vi "Scope_V3.vi"(9 "ObjectChoice":i32[](listbox), 11 "btnSelectObject":bool) -> (0 "strObjectDispArray":string[](array[string]), 1 "mu08ArrayIndexFinalOut":u8[](array[numeric]), 2 "NamePic":picture, 3 "mbfObjectChoiceArray":bool[](array[boolean]))   [LabVIEW 2011]
uses:
  <vilib>/Utility/miscctls.llb/LVPoint32TypeDef.ctl
  GlobalVariable/strGlobalVariable.vi
panel:
  out "mbfStartDraw":bool
  out "btnSelectObject.Txt":string
  out "坐标":T1
  out "mu08ObjectArraySize":u8
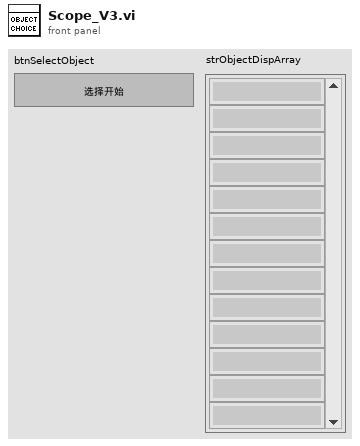
[diagram p1: front panel]
types:
  T1 = typedef "LVPoint32TypeDef.ctl" = cluster{"Horizontal":i32, "Vertical":i32}
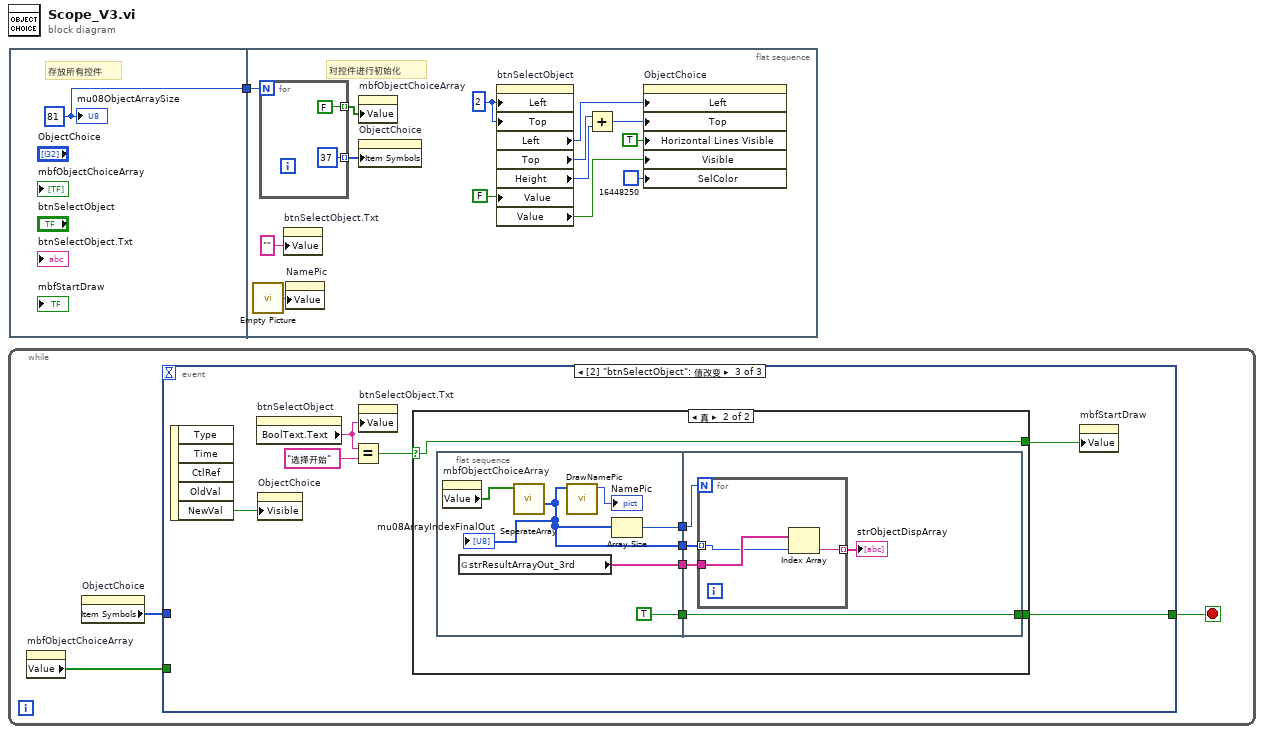
[diagram p0: block diagram]
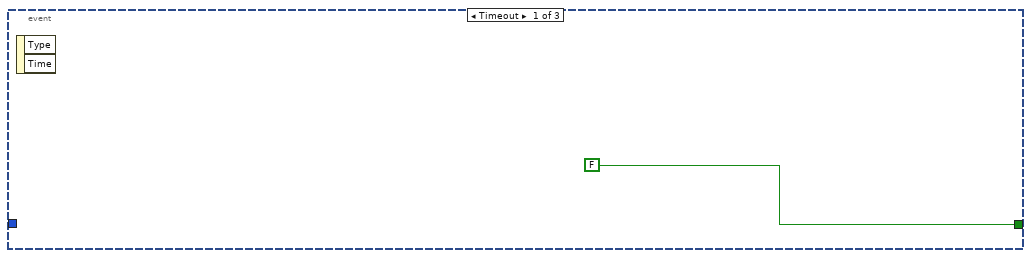
[diagram p2: hidden frame]
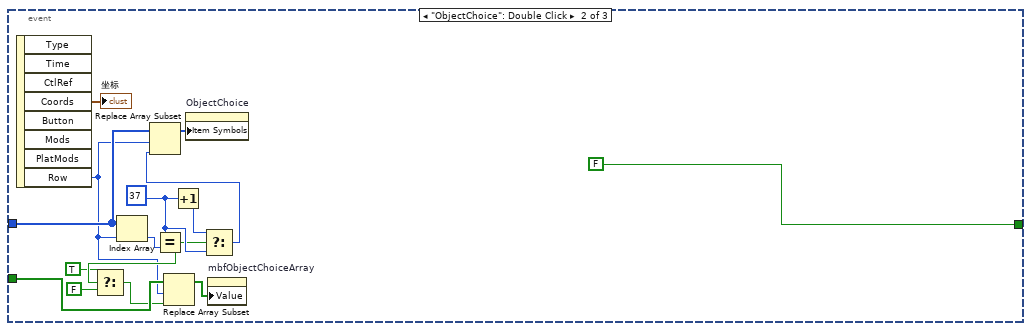
[diagram p3: hidden frame]
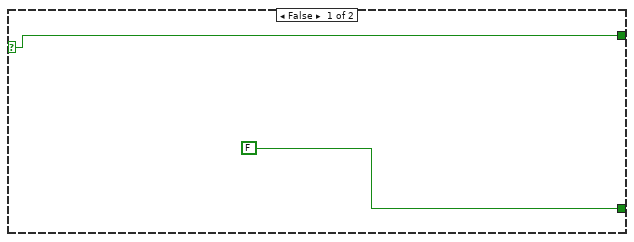
[diagram p4: hidden frame]
diagram:
  n1 = while {
    stop <- w2 stop-if-true
    n2 = property on="mbfObjectChoiceArray" class="Arr (严格)"() -> ("Value"=w3:bool[])  [unwired: 2 in, 2 out]
    n3 = property on="ObjectChoice" class="LstBox (严格)"() -> ("Item Symbols"=w4:i32[])  [unwired: 2 in, 2 out]
    n4 = event shown="[2] \"btnSelectObject\": 值改变" {
      selector: _ -> [_ _ _]
      dyn-events: _ -> [_ _ _]
      timeout: _ -> [_ _ _]
      tunnel: w4 -> [_ w19 _]
      tunnel: w3 -> [_ w10 _]
      tunnel: [FALSE FALSE w21] -> w2
      event Timeout {
        n5 = event-data() -> ()  [unwired: 1 in, 2 out]
      }
      event "ObjectChoice": Double Click {
        w15 = 37 ("y")
        n6 = event-data() -> ("Coords"=→"坐标":T1, "Row"=w7:i32)  [unwired: 1 in, 6 out]
        n7 = Index Array(array=w19, index=w7) -> (element=w17:i32)
        n8 = Equal?(x=w15, y=w17) -> (x = y?=w13:bool)
        n9 = Select(t=TRUE, s=w13, f=FALSE) -> (s? t:f=w9:bool)
        n10 = Replace Array Subset(array=w10, new element=w9, index=w7) -> (w8:bool[])
        n11 = Increment(x=w15) -> (x+1=w16:i32)
        n12 = Select(t=w16, s=w13, f=w15) -> (s? t:f=w14:i32)
        n13 = Replace Array Subset(array=w19, new element=w14, index=w7) -> (w18:i32[])
        n14 = property on="ObjectChoice" class="LstBox (严格)"("Item Symbols"=w18) -> ()  [unwired: 2 in, 2 out]
        n15 = property on="mbfObjectChoiceArray" class="Arr (严格)"("Value"=w8) -> ()  [unwired: 2 in, 2 out]
      }
      event "btnSelectObject": Value Change {
        n16 = event-data() -> ("NewVal"=w26:bool)  [unwired: 1 in, 4 out]
        n17 = property on="btnSelectObject" class="Bool (严格)"() -> ("BoolText.Text"=w25:string)  [unwired: 2 in, 2 out]
        n18 = property on="ObjectChoice" class="LstBox (严格)"("Visible"=w26) -> ()  [unwired: 2 in, 2 out]
        n19 = Equal?(x=w25, y="选择开始") -> (x = y?=w23:bool)
        n20 = property on="btnSelectObject.Txt" class="Str"("Value"=w25) -> ()  [unwired: 2 in, 2 out]
        n21 = case shown="真" w23 {
          selector: w23 -> [w28 w34]
          tunnel: [w28 w34] -> w22
          tunnel: [FALSE w33] -> w21
          frame False {
          }
          frame True {
            n22 = flat-sequence {
              tunnel: [TRUE] -> w32
              tunnel: [w37] -> w31
              tunnel: [w35] -> w30
              tunnel: [w36] -> w29
              tunnel: [w45] -> w33
              tunnel: w32 -> [w45]
              tunnel: w31 -> [w44]
              tunnel: w30 -> [w43]
              tunnel: w29 -> [w42]
              frame #0 {
                n23 = property on="mbfObjectChoiceArray" class="Arr (严格)"() -> ("Value"=w40:bool[])  [unwired: 2 in, 2 out]
                n24 = global read "strGlobalVariable.vi" "strResultArrayOut_3rd"() -> (w35:string[])
                n25 = call "SeperateArray.vi"("mbfArrayIn"=w40) -> ("mu08ArrayIndexFinalOut"=w36:u8[])  [unwired: 9 in, 1 out]
                "mu08ArrayIndexFinalOut" <- w36
                n26 = call "DrawNamePic.vi"("mu08ArrayIn"=w36) -> ("NamePic"=→"NamePic":picture)  [unwired: 10 in]
                n27 = Array Size(array=w36) -> (size(s)=w37:i32)
              }
              frame #1 {
                n28 = for {
                  N: w44 -> [_]
                  tunnel: w43 -> [w48]
                  tunnel: w42 -> [w47] mode=indexing
                  tunnel: [w46] -> w41 mode=indexing
                  n29 = Index Array(array=w48, index=w47) -> (element=w46:string)
                }
                "strObjectDispArray" <- w41
              }
            }
          }
        }
        n30 = property on="mbfStartDraw" class="Bool (严格)"("Value"=w22) -> ()  [unwired: 2 in, 2 out]
      }
    }
  }
  n31 = flat-sequence {
    tunnel: [w49] -> w1
    tunnel: w1 -> [w63]
    frame #0 {
      w49 = u8 81 ("mu08ObjectArraySize")
      # "存放所有控件"
      "mu08ObjectArraySize" <- w49
    }
    frame #1 {
      w55 = 2 ("位置:居左")
      # "对控件进行初始化"
      n32 = call "Empty Picture"() -> ("empty picture"=w50:picture)
      n33 = for {
        N: w63 -> [_]
        tunnel: [FALSE] -> w61 mode=indexing
        tunnel: [37] -> w62 mode=indexing
      }
      n34 = property on="btnSelectObject.Txt" class="Str"("Value"="" ("btnSelectObject.Txt")) -> ()  [unwired: 2 in, 2 out]
      n35 = property on="NamePic" class="Pict"("Value"=w50) -> ()  [unwired: 2 in, 2 out]
      n36 = property on="mbfObjectChoiceArray" class="Arr (严格)"("Value"=w61) -> ()  [unwired: 2 in, 2 out]
      n37 = property on="ObjectChoice" class="LstBox (严格)"("Item Symbols"=w62) -> ()  [unwired: 2 in, 2 out]
      n38 = property on="btnSelectObject" class="Bool (严格)"("Left"=w55, "Top"=w55, "Value"=FALSE ("btnSelectObject")) -> ("Left"=w60:i32, "Top"=w53:i32, "Height"=w59:u32, "Value"=w54:bool)  [unwired: 2 in, 2 out]
      n39 = Add(x=w53, y=w59) -> (x+y=w58:u32)
      n40 = property on="ObjectChoice" class="LstBox (严格)"("Left"=w60, "Top"=w58, "Horizontal Lines Visible"=TRUE, "Visible"=w54, "SelColor"=u32 16448250) -> ()  [unwired: 2 in, 2 out]
    }
  }
